vi "PathPlanner.vi"(11 "IA State Output in":T1) -> (3 "IA State Output out":T1)   [LabVIEW 2017]
uses:
  Core/AI Input.ctl
  Core/AI Robot.ctl
  Intel/Functions Enum.ctl
  Intel/AttackerStates.ctl
  RRT/PathDests.ctl
  RRT/PathDest.ctl
  Core/AI Ball.ctl
  Core/Field Size.ctl
  Core/AI Judge.ctl
  Intel/Command Enum.ctl
  Util/Events/Events.ctl
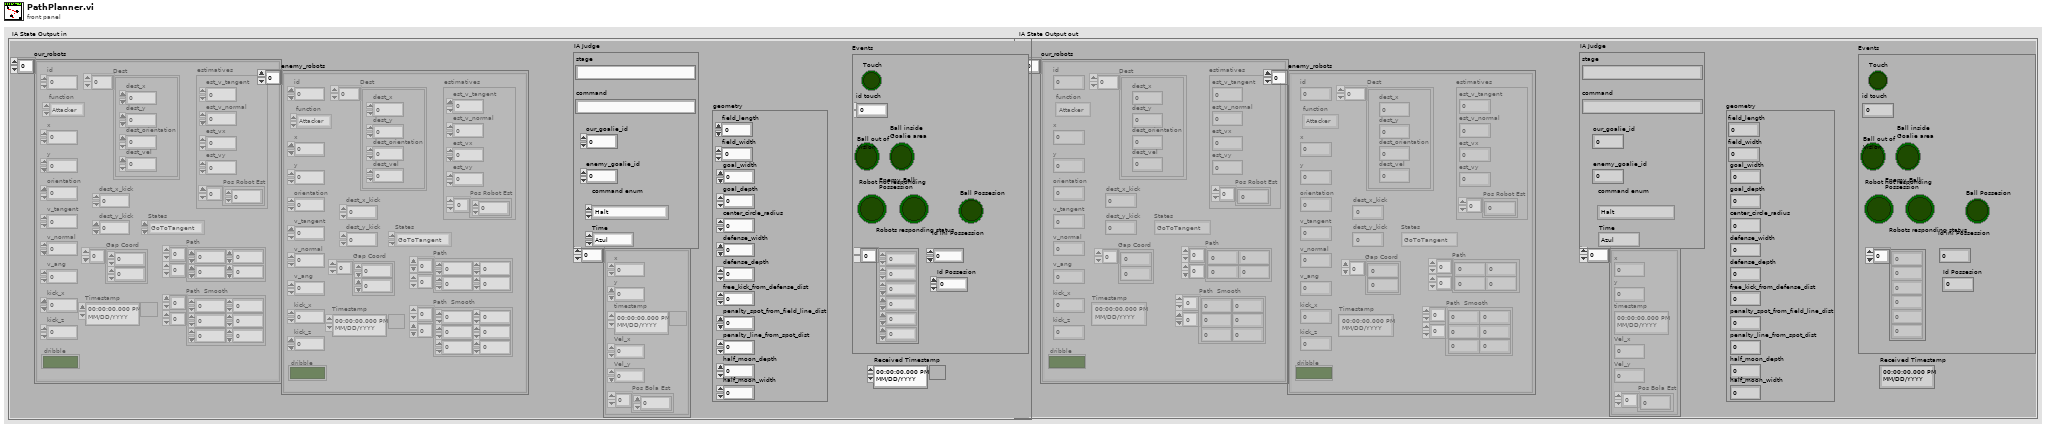
[diagram p1: front panel]
types:
  T1 = typedef "AI Input.ctl" = cluster{"our_robots":T2[], "enemy_robots":T2[], "balls":T7[], "geometry":T8, "IA Judge":T9, "Received Timestamp":timestamp, "Events":T11}
  T2 = typedef "AI Robot.ctl" = cluster{"id":u32, "function":T3, "x":dbl, "y":dbl, "orientation":dbl, "v_tangent":dbl, "v_normal":dbl, "v_ang":dbl, "kick_x":dbl, "kick_z":dbl, "dribble":bool, "Timestamp":timestamp, "estimatives":cluster{"est_v_tangent":dbl, "est_v_normal":dbl, "est_vx":dbl, "est_vy":dbl, "Pos Robot Est":dbl[]}, "dest_x_kick":dbl, "dest_y_kick":dbl, "Gap Coord":dbl[], "States":T4, "Path ":dbl[][], "Path  Smooth":dbl[][], "Dest":T5}
  T3 = typedef "Functions Enum.ctl" = enum16{"Attacker", "Goalie", "Defender", "Striker", "Goto 0", "Dummy", "Kicker", "ZigZag"}
  T4 = typedef "AttackerStates.ctl" = enum16{"Pass", "GoToTangent", "BallGetting", "GoToKick", "Rotate anti-clockwise", "Rotate Clockwise", ""}
  T5 = typedef "PathDests.ctl" = T6[]
  T6 = typedef "PathDest.ctl" = cluster{"dest_x":dbl, "dest_y":dbl, "dest_orientation":dbl, "dest_vel":dbl}
  T7 = typedef "AI Ball.ctl" = cluster{"x":dbl, "y":dbl, "timestamp":timestamp, "Vel_x":dbl, "Vel_y":dbl, "Pos Bola Est":dbl[]}
  T8 = typedef "Field Size.ctl" = cluster{"field_length":u32, "field_width":u32, "goal_width":u32, "goal_depth":u32, "center_circle_radius":u32, "defense_width":u32, "defense_depth":u32, "free_kick_from_defense_dist":u32, "penalty_spot_from_field_line_dist":u32, "penalty_line_from_spot_dist":u32, "half_moon_depth":u32, "half_moon_width":u32}
  T9 = typedef "AI Judge.ctl" = cluster{"stage":string, "command":string, "our_goalie_id":dbl, "enemy_goalie_id":dbl, "command enum":T10, "Time":enum16{"Azul", "Amarelo"}}
  T10 = typedef "Command Enum.ctl" = enum16{"Halt", "Stop", "Force Start", "PKA Normal Start", "Prepare Kickoff Ally", "PKE Normal Start", "Prepare Kickoff Enemy", "Prepare Penalty Ally", "PPA Normal Start", "Prepare Penalty Enemy", "PPE Normal Start", "Direct Free Enemy", "Direct Free Ally", "Indirect Free Enemy", "Indirect Free Ally", "Timeout Enemy", "Timeout Ally", "Goal Enemy", "Goal Ally", "Ball Placement Enemy", "Ball Placement Ally", "Normal Half Time", "Extra Time Break", "Extra Half Time", "None", "Post Game"}
  T11 = typedef "Events.ctl" = cluster{"Touch":bool, "id touch":dbl, "Ball out of \nVision":bool, "Ball inside \nGoalie area":bool, "Robot not responding":bool, "Robots responding status":dbl[], "Enemy Ball \nPossession":bool, "Id ini Possession":dbl, "Ball Possesion":bool, "Id Possesion":dbl}
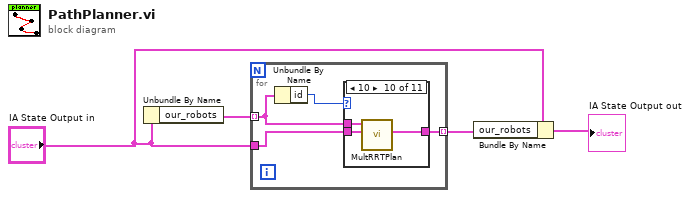
[diagram p0: block diagram]
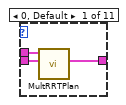
[diagram p2: hidden frame]
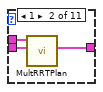
[diagram p3: hidden frame]
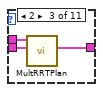
[diagram p4: hidden frame]
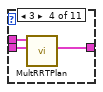
[diagram p5: hidden frame]
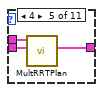
[diagram p6: hidden frame]
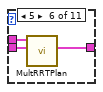
[diagram p7: hidden frame]
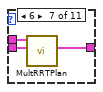
[diagram p8: hidden frame]
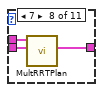
[diagram p9: hidden frame]
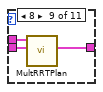
[diagram p10: hidden frame]
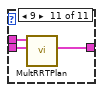
[diagram p11: hidden frame]
diagram:
  n1 = Unbundle By Name("IA State Output in") -> ("our_robots"=w1:T2[])
  n2 = for {
    tunnel: "IA State Output in" -> [w8]
    tunnel: w1 -> [w6] mode=indexing
    tunnel: [w7] -> w2 mode=indexing
    n3 = Unbundle By Name(w6) -> ("id"=w5:u32)
    n4 = case shown="10" w5 {
      tunnel: w8 -> [w11 w14 w17 w20 w23 w26 w29 w32 w35 w38 w41]
      tunnel: [w9 w12 w15 w18 w21 w24 w27 w30 w33 w36 w39] -> w7
      tunnel: w6 -> [w10 w13 w16 w19 w22 w25 w28 w31 w34 w37 w40]
      frame 0, Default {
        n5 = call "MultRRTPlan.vi"("IA State"=w11, "Robot"=w10) -> ("Robot Out"=w9:T2)  [unwired: 9 in]
      }
      frame 1 {
        n6 = call "MultRRTPlan.vi"("IA State"=w14, "Robot"=w13) -> ("Robot Out"=w12:T2)  [unwired: 9 in]
      }
      frame 2 {
        n7 = call "MultRRTPlan.vi"("IA State"=w17, "Robot"=w16) -> ("Robot Out"=w15:T2)  [unwired: 9 in]
      }
      frame 3 {
        n8 = call "MultRRTPlan.vi"("IA State"=w20, "Robot"=w19) -> ("Robot Out"=w18:T2)  [unwired: 9 in]
      }
      frame 4 {
        n9 = call "MultRRTPlan.vi"("IA State"=w23, "Robot"=w22) -> ("Robot Out"=w21:T2)  [unwired: 9 in]
      }
      frame 5 {
        n10 = call "MultRRTPlan.vi"("IA State"=w26, "Robot"=w25) -> ("Robot Out"=w24:T2)  [unwired: 9 in]
      }
      frame 6 {
        n11 = call "MultRRTPlan.vi"("IA State"=w29, "Robot"=w28) -> ("Robot Out"=w27:T2)  [unwired: 9 in]
      }
      frame 7 {
        n12 = call "MultRRTPlan.vi"("IA State"=w32, "Robot"=w31) -> ("Robot Out"=w30:T2)  [unwired: 9 in]
      }
      frame 8 {
        n13 = call "MultRRTPlan.vi"("IA State"=w35, "Robot"=w34) -> ("Robot Out"=w33:T2)  [unwired: 9 in]
      }
      frame 10 {
        n14 = call "MultRRTPlan.vi"("IA State"=w38, "Robot"=w37) -> ("Robot Out"=w36:T2)  [unwired: 9 in]
      }
      frame 9 {
        n15 = call "MultRRTPlan.vi"("IA State"=w41, "Robot"=w40) -> ("Robot Out"=w39:T2)  [unwired: 9 in]
      }
    }
  }
  n16 = Bundle By Name(cluster="IA State Output in", "our_robots"=w2) -> (→"IA State Output out":T1)
